vi "WLAN - niVST - RFSA - Gain and Trigger Settings.vi"(0 "instrument handle":refnum<k15>, 7 "External Attenuation (dB)":dbl, 11 "error in":errorcluster) -> (4 "instrument handle":refnum<k15>, 15 "error out":errorcluster)   [LabVIEW 2012]
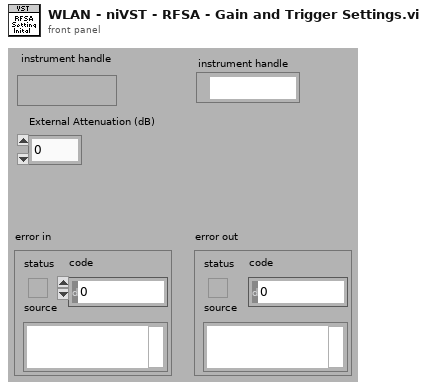
[diagram p1: front panel]
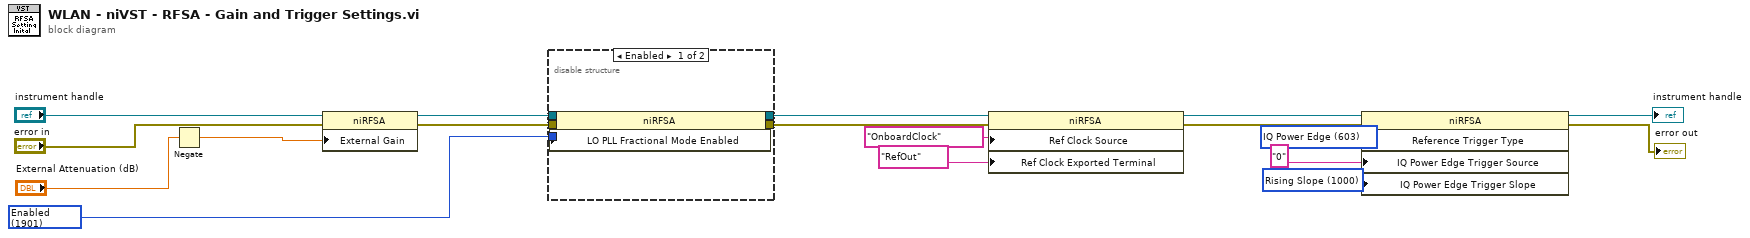
[diagram p0: block diagram]
diagram:
  w11 = 1000 items=["Rising Slope"=1000, "Falling Slope"=1001] ("Triggers:Ref:IQ Power Edge:Slope")
  w13 = 603 items=["None"=600, "Digital Edge"=601, "IQ Power Edge"=603, "Software"=604, "IQ Analog Edge"=605] ("Triggers:Ref:Type")
  w2 = 1901 items=["Disabled"=1900, "Enabled"=1901] ("RF-RIO:Signal Path:LO PLL Fractional Mode Enabled")
  n1 = Negate(x="External Attenuation (dB)") -> (-x=w15:dbl)
  n2 = property on="Property Node" class="niRFSA"(reference="instrument handle", error in="error in", "External Gain"=w15) -> (reference out=w6:refnum<k15>, error out=w3:errorcluster)
  n3 = disable-structure shown="Enabled" {
    disable-tunnel: w6 -> [w23 w24]
    disable-tunnel: [w22 w24] -> w5
    disable-tunnel: [w21 w25] -> w4
    disable-tunnel: w3 -> [w20 w25]
    disable-tunnel: w2 -> [w19 _]
    frame Enabled {
      n4 = property on="Property Node" class="niRFSA"(reference=w23, error in=w20, "LO PLL Fractional Mode Enabled"=w19) -> (reference out=w22:refnum<k15>, error out=w21:errorcluster)
    }
    frame Disabled {
    }
  }
  n5 = property class="niRFSA"(reference=w5, error in=w4, "Ref Clock Source"="OnboardClock" ("Clocking:Ref Clock Source"), "Ref Clock Exported Terminal"="RefOut" ("Clocking:Ref Clock Exported Terminal")) -> (reference out=w10:refnum<k15>, error out=w9:errorcluster)
  n6 = property class="niRFSA"(reference=w10, error in=w9, "Reference Trigger Type"=w13, "IQ Power Edge Trigger Source"="0" ("source"), "IQ Power Edge Trigger Slope"=w11) -> (reference out=→"instrument handle":refnum<k15>, error out=→"error out":errorcluster)
